vi "Util_SpeedDividerMath.vi"(11 "Axis Value":dbl) -> (3 "Divider Value":dbl)   [LabVIEW 2017]
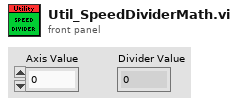
[diagram p1: front panel]
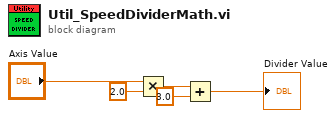
[diagram p0: block diagram]
diagram:
  n1 = Multiply(x="Axis Value", y=2.0) -> (x*y=w2:dbl)
  n2 = Add(x=w2, y=3.0) -> (x+y=→"Divider Value":dbl)
